vi "Register Value.vi"(10 "Register":i32, 11 "Registers":T1[](array[typedef]) format="%032b") -> (3 "Platter":T1 format="%032b")   [LabVIEW 2020]
uses:
  Platter.ctl
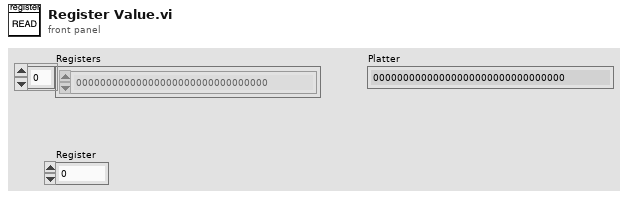
[diagram p1: front panel]
types:
  T1 = typedef "Platter.ctl" = u32
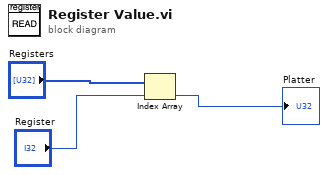
[diagram p0: block diagram]
diagram:
  n1 = Index Array(array="Registers", index="Register") -> (element=→"Platter":T1)
